vi "Pololu.Mgr - Set VID, PID.vi"(8 "error in (no error)":errorcluster, 11 "PololuCtrl in":refnum<class "PololuCtrl.lvclass">) -> (0 "error out":errorcluster, 3 "PololuCtrl out":refnum<class "PololuCtrl.lvclass">)   [LabVIEW 2018, in "PololuCtrl.lvclass"]
uses:
  PololuCtrl.lvclass
  PololuCtrl.lvclass/PololuCtrl.ctl
panel:
  in  "PID":string
  in  "VID":string
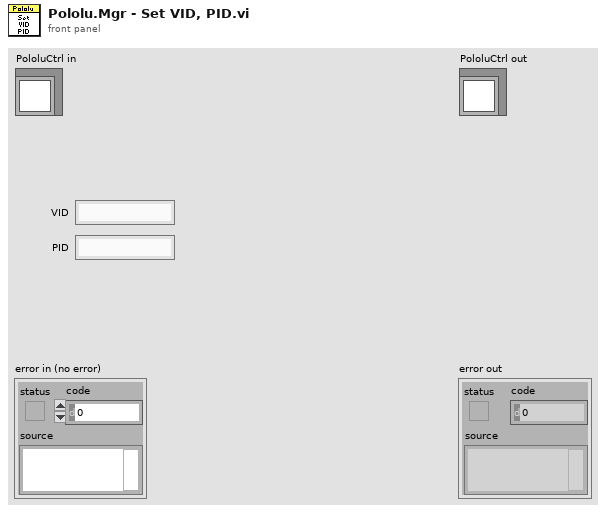
[diagram p1: front panel]
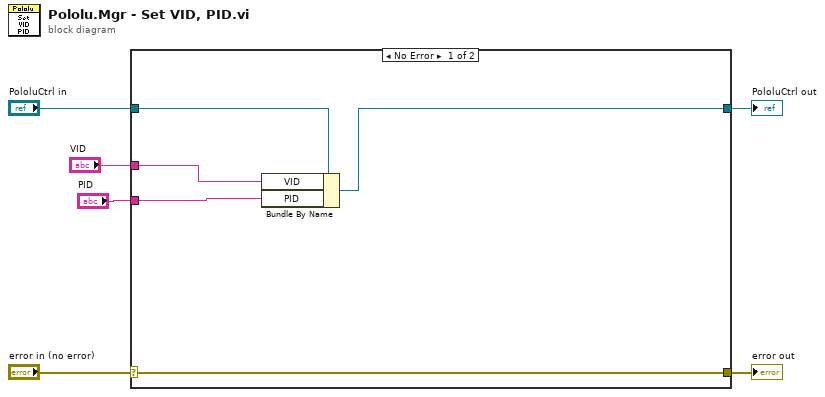
[diagram p0: block diagram]
diagram:
  n1 = case shown="No Error" "error in (no error)" {
    selector: "error in (no error)" -> [w11 w13]
    tunnel: [w11 w13] -> w5
    tunnel: [w8 w12] -> w3
    tunnel: "PololuCtrl in" -> [w7 w12]
    tunnel: "VID" -> [w10 _]
    tunnel: "PID" -> [w9 _]
    frame No Error {
      n2 = Bundle By Name(cluster=w7, "VID"=w10, "PID"=w9) -> (w8:refnum<class "PololuCtrl.lvclass">)
    }
    frame Error {
    }
  }
  "error out" <- w5
  "PololuCtrl out" <- w3
